vi "EMV PI Controller.vi"(8 "error in (no error)":errorcluster, 11 "Error":dbl) -> (0 "error out":errorcluster, 3 "PI Saturated":bool)   [LabVIEW 2020]
panel:
  out "x >> y 2":i32
  in  "Kp Qbits Value 2":i32
  in  "Error":i16
  in  "Kp Gain Value 2":i16
  in  "y 2":i16
  in  "x 2":i16
  out "x2 >> y 2":i16
  out "x << y":i16
  in  "x":i16
  in  "y":i16
  in  "Kp Gain Value":i32
  in  "Kp Qbits Value":i32
  in  "Ki Gain Value":i32
  in  "Ki Qbits Value":i32
  out "I Value":dbl min=40.0 max=190.0 step=1.0
  out "P Value":dbl min=40.0 max=190.0 step=1.0
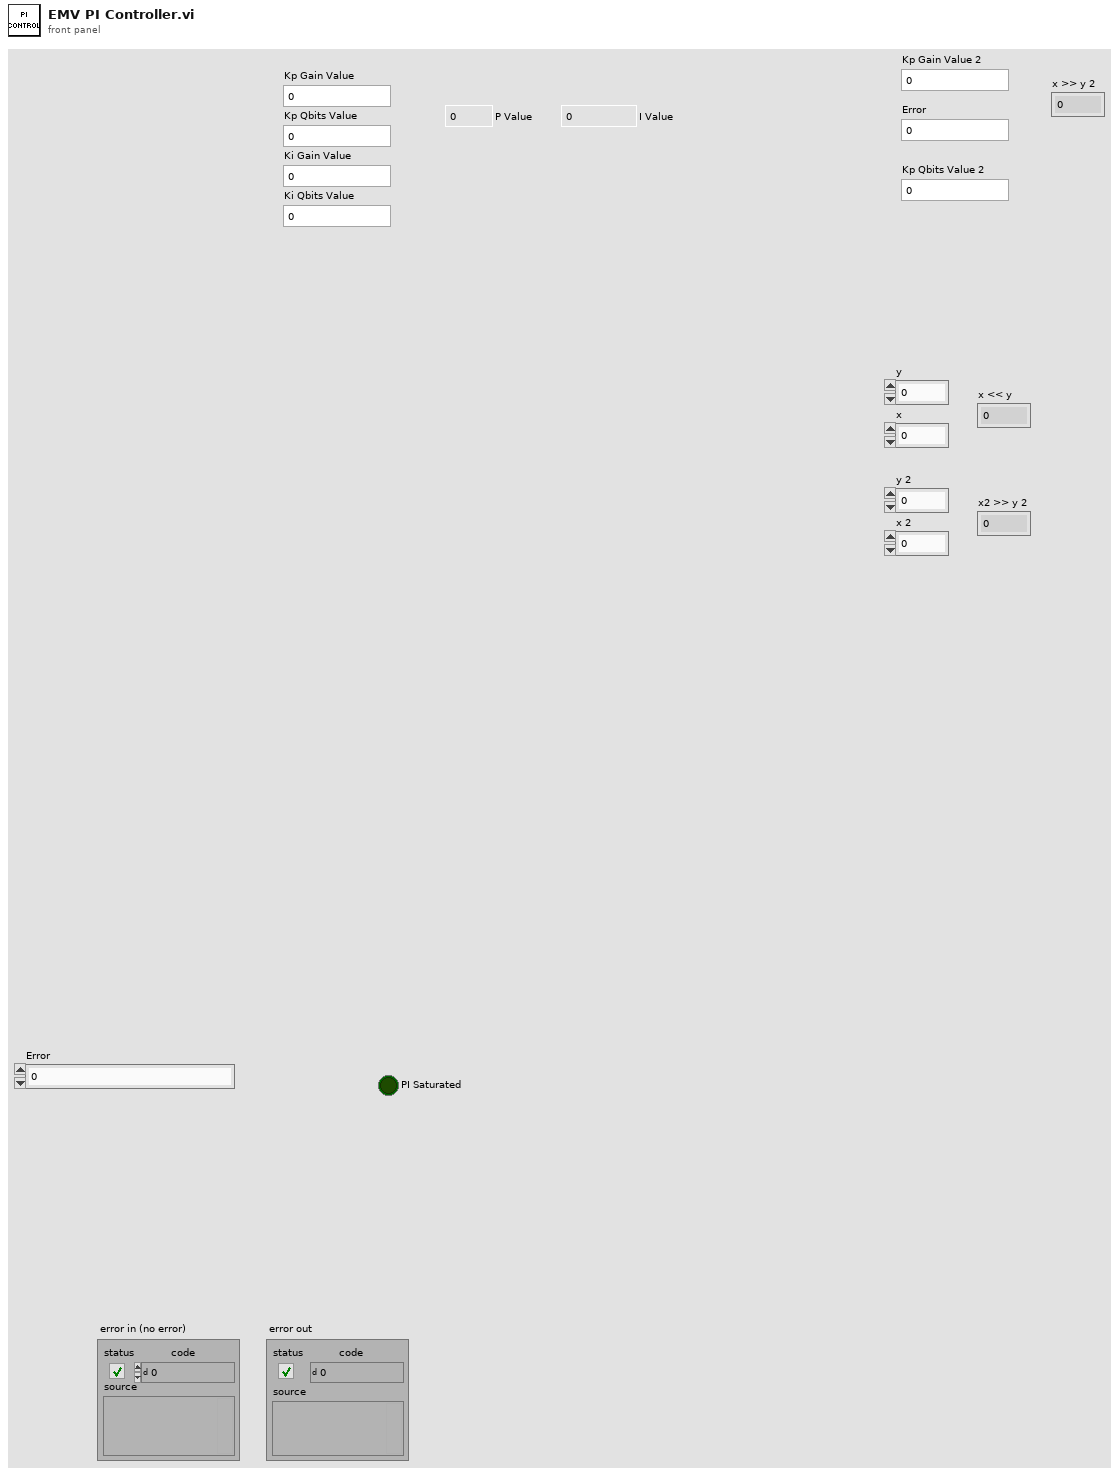
[diagram p1: front panel]
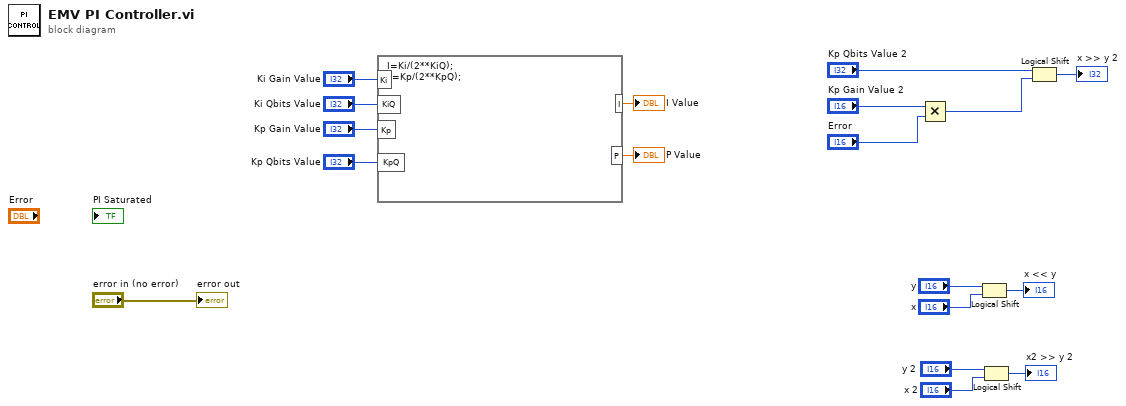
[diagram p0: block diagram]
diagram:
  n1 = formula code="I=Ki/(2**KiQ);\nP=Kp/(2**KpQ);"("Ki"="Ki Gain Value", "KiQ"="Ki Qbits Value", "Kp"="Kp Gain Value", "KpQ"="Kp Qbits Value") -> ("I"=→"I Value":dbl, "P"=→"P Value":dbl)
  n2 = Multiply(x="Kp Gain Value 2", y="Error") -> (x*y=w1:i16)
  n3 = Logical Shift(y="y", x="x") -> (x << y=→"x << y":i16)
  n4 = Logical Shift(y="y 2", x="x 2") -> (x << y=→"x2 >> y 2":i16)
  n5 = Logical Shift(y="Kp Qbits Value 2", x=w1) -> (x << y=→"x >> y 2":i16)
  "error out" <- "error in (no error)"
